vi "Check Homing Status V2.vi"(6 "Ignore Limit Switches?":bool, 7 "Prev Encoder":i32, 8 "error in (no error)":errorcluster, 9 "Status Byte in":u8, 10 "Homing Count in":i32, 11 "New Encoder":i32) -> (0 "error out":errorcluster, 2 "Homing Count Out":i32, 3 "Home Complete":bool)   [LabVIEW 2015, in "Tool Module.lvlib"]
uses:
  Tool Module.lvlib
  ToolModGLOB.vi
  <vilib>/Utility/error.llb/Error Cluster From Error Code.vi
  <vilib>/ErrorRing/Error Ring.xnode
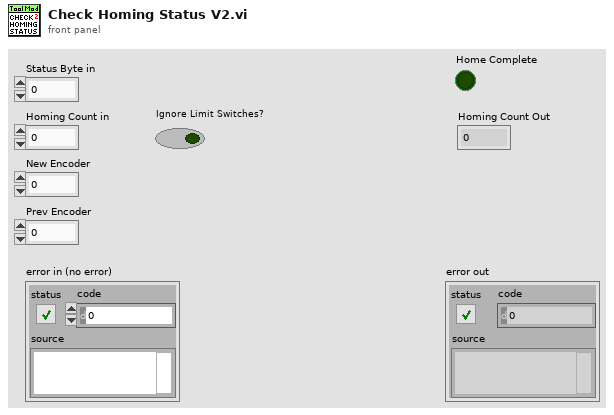
[diagram p1: front panel]
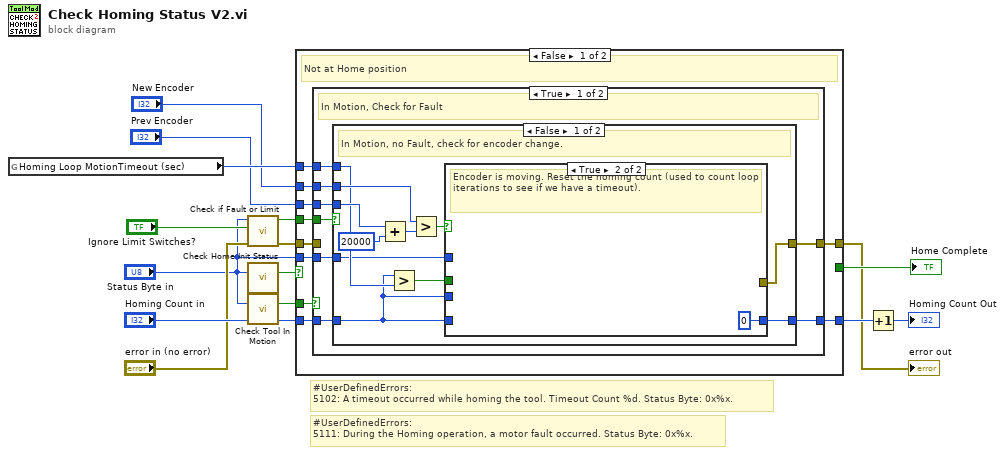
[diagram p0: block diagram]
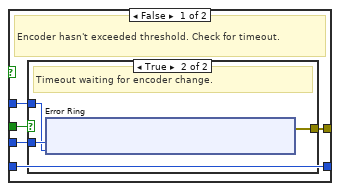
[diagram p2: hidden frame]
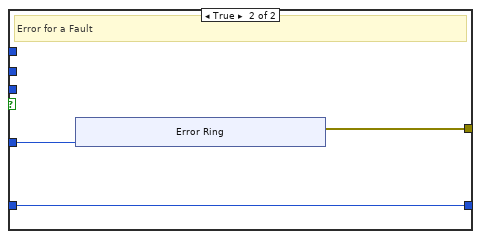
[diagram p4: hidden frame]
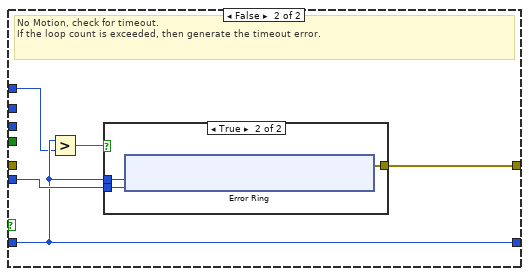
[diagram p5: hidden frame]
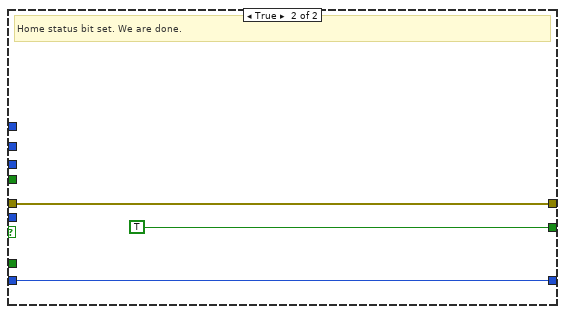
[diagram p7: hidden frame]
diagram:
  # "#UserDefinedErrors:\n5102: A timeout occurred while homing the tool. Timeout Count %d. Status Byte: 0x%x."
  # "#UserDefinedErrors:\n5111: During the Homing operation, a motor fault occurred. Status Byte: 0x%x."
  n1 = global read "ToolModGLOB.vi" "Homing Loop MotionTimeout (sec)"() -> (w5:i32)
  n2 = call "Check if Fault or Limit.vi"("error in (no error)"="error in (no error)", "Ignore Limit Switches?"="Ignore Limit Switches?", "Status In"="Status Byte in") -> ("error out"=w13:errorcluster, "Fault or Limit"=w14:bool)  [unwired: 7 in]
  n3 = call "Check Home Init Status.vi"("Status Byte"="Status Byte in") -> ("Home Init?"=w15:bool)  [unwired: 14 in]
  n4 = call "Check Tool In Motion.vi"("Status Byte"="Status Byte in") -> ("Tool In Motion?"=w3:bool)  [unwired: 14 in]
  n5 = case shown="False" w15 {
    tunnel: w14 -> [w18 _]
    tunnel: [w25 w89] -> w6
    tunnel: [_ TRUE] -> w12
    tunnel: w13 -> [w24 w89]
    tunnel: "Status Byte in" -> [w23 _]
    tunnel: "Homing Count in" -> [w22 w88]
    tunnel: [w21 w88] -> w8
    tunnel: w5 -> [w20 _]
    tunnel: w3 -> [w19 _]
    tunnel: "New Encoder" -> [w17 _]
    tunnel: "Prev Encoder" -> [w16 _]
    frame False {
      # "Not at Home position"
      n6 = case shown="True" w19 {
        tunnel: [w33 w75] -> w25
        tunnel: w24 -> [_ _]
        tunnel: w23 -> [w32 w76]
        tunnel: w22 -> [w28 w74]
        tunnel: [w26 w74] -> w21
        tunnel: w20 -> [w27 w73]
        tunnel: w18 -> [w31 _]
        tunnel: w17 -> [w30 _]
        tunnel: w16 -> [w29 _]
        frame True {
          # "In Motion, Check for Fault"
          n7 = case shown="False" w31 {
            tunnel: [w37 w64] -> w33
            tunnel: w32 -> [w36 w63]
            tunnel: w30 -> [w43 _]
            tunnel: w29 -> [w42 _]
            tunnel: w28 -> [w35 w62]
            tunnel: w27 -> [w39 _]
            tunnel: [w34 w62] -> w26
            frame False {
              # "In Motion, no Fault, check for encoder change."
              n8 = Add(x=w42, y=20000) -> (x+y=w40:i32)
              n9 = Greater?(x=w35, y=w39) -> (0:w38:bool)
              n10 = Greater?(x=w43, y=w40) -> (0:w44:bool)
              n11 = case shown="True" w44 {
                tunnel: w38 -> [w49 _]
                tunnel: [w48 _] -> w37
                tunnel: w35 -> [w47 _]
                tunnel: w36 -> [w46 _]
                tunnel: w35 -> [w45 _]
                tunnel: [w45 0 ("Homing Count in")] -> w34
                frame False {
                  # "Encoder hasn't exceeded threshold. Check for timeout."
                  n12 = case shown="True" w49 {
                    tunnel: [_ w52] -> w48
                    tunnel: w47 -> [_ w51]
                    tunnel: w46 -> [_ w50]
                    frame False {
                    }
                    frame True {
                      # "Timeout waiting for encoder change."
                      n13 = xnode "Error Ring"("parameter 0"=w51, "parameter 1"=w50) -> ("error out"=w52:errorcluster)
                    }
                  }
                }
                frame True {
                  # "Encoder is moving. Reset the homing count (used to count loop iterations to see if we have a timeout)."
                }
              }
            }
            frame True {
              # "Error for a Fault"
              n14 = xnode "Error Ring"("parameter 0"=w63) -> ("error out"=w64:errorcluster)
            }
          }
        }
        frame False {
          # "No Motion, check for timeout.\nIf the loop count is exceeded, then generate the timeout error."
          n15 = Greater?(x=w74, y=w73) -> (0:w72:bool)
          n16 = case shown="True" w72 {
            tunnel: [_ w79] -> w75
            tunnel: w76 -> [_ w78]
            tunnel: w74 -> [_ w77]
            frame False {
            }
            frame True {
              n17 = xnode "Error Ring"("parameter 0"=w77, "parameter 1"=w78) -> ("error out"=w79:errorcluster)
            }
          }
        }
      }
    }
    frame True {
      # "Home status bit set. We are done."
    }
  }
  "error out" <- w6
  "Home Complete" <- w12
  n18 = Increment(x=w8) -> (x+1=→"Homing Count Out":i32)
